vi "vms_issueCommand_enterControl.vi"(8 "error in (no error)":errorcluster, 11 "command_enterControl_Ctl":T1) -> (0 "error out":errorcluster, 2 "function return":i32, 3 "command_enterControl_Ctl out":T1)   [LabVIEW 2016, in "SALLV_vms.lvlib"]
doc: "int vms_shm_issueCommand_enterControlLV(vms_command_enterControlLV *command_enterControl_Ctl );"
uses:
  SALLV_vms.lvlib
  DataTypes/command_enterControl.ctl
  SALLV_vms.so
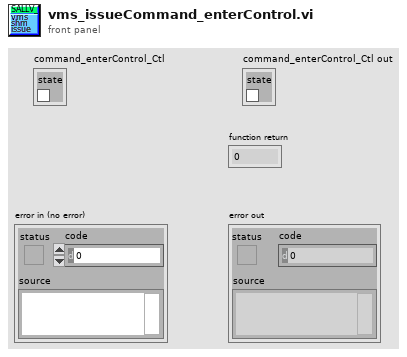
[diagram p1: front panel]
types:
  T1 = typedef "SALLV_vms.lvlib/command_enterControl.ctl" = cluster{"state":bool}
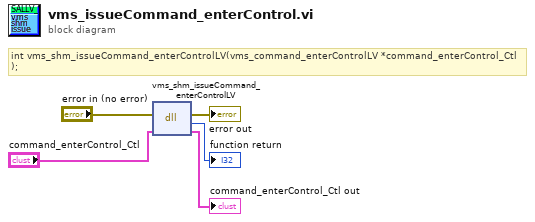
[diagram p0: block diagram]
diagram:
  # "int vms_shm_issueCommand_enterControlLV(vms_command_enterControlLV *command_enterControl_Ctl );"
  n1 = dll-call lib="opt/CODE/SALLV_vms/SALLV_vms.*" fn="vms_shm_issueCommand_enterControlLV"(error in="error in (no error)", "command_enterControl_Ctl"="command_enterControl_Ctl") -> (error out=→"error out":errorcluster, →"function return":i32, "command_enterControl_Ctl"=→"command_enterControl_Ctl out":T1)  [unwired: 2 in, 1 out]
